vi "Get FP Window Handle.vi"(8 "错误输入（无错误）":errorcluster, 11 "VI Ref In":refnum<vi>) -> (0 "错误输出":errorcluster, 2 "VIRef.lvlib:Window Refnum":T1, 3 "VI Ref Out":refnum<vi>)   [LabVIEW 2012, in "VIRef.lvlib"]
uses:
  VIRef.lvlib
  Window Refnum.ctl
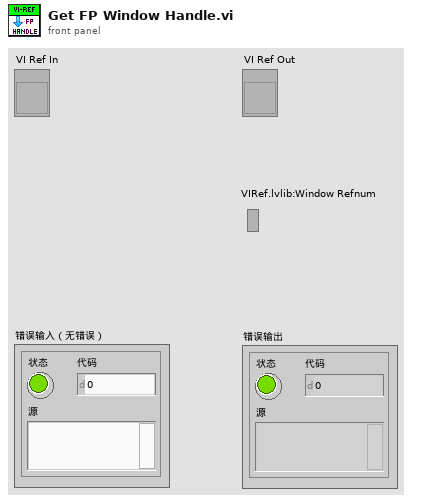
[diagram p1: front panel]
types:
  T1 = typedef "VIRef.lvlib/Window Refnum.ctl" = refnum<k1>
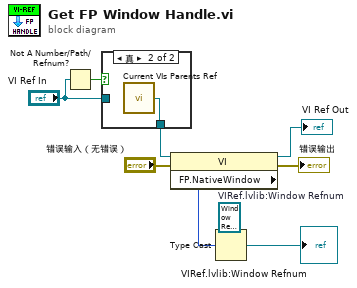
[diagram p0: block diagram]
diagram:
  w2 = T1 refnum  # VIRef.lvlib:Window Refnum
  n1 = Not A Number/Path/Refnum?(number/path/refnum="VI Ref In") -> (NaN/Path/Refnum?=w9:bool)
  n2 = case shown="真" w9 {
    tunnel: [w10 w11] -> w4
    tunnel: "VI Ref In" -> [w10 _]
    frame False {
    }
    frame True {
      n3 = call "Current VIs Parents Ref.vi"() -> ("Calling VI's Reference"=w11:refnum<vi>)  [unwired: 2 in]
    }
  }
  n4 = property class="VI"(reference=w4, error in="错误输入（无错误）") -> (reference out=→"VI Ref Out":refnum<vi>, error out=→"错误输出":errorcluster, "FP.NativeWindow"=w3:u64)
  n5 = Type Cast(type=w2, x=w3) -> (*(type *) &x=→"VIRef.lvlib:Window Refnum":T1)
